vi "SampleRelativeMove.vi"() -> ()   [LabVIEW 2012]
panel:
  in  "Relative Steps":i32=15000
  in  "Motor Number":i32=1
  in  "stop":bool
  out "Position Status":i32
  out "error out":errorcluster
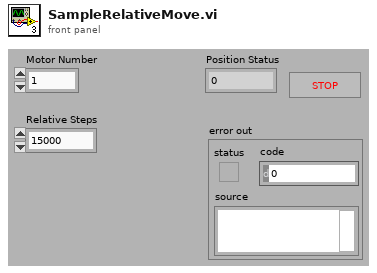
[diagram p1: front panel]
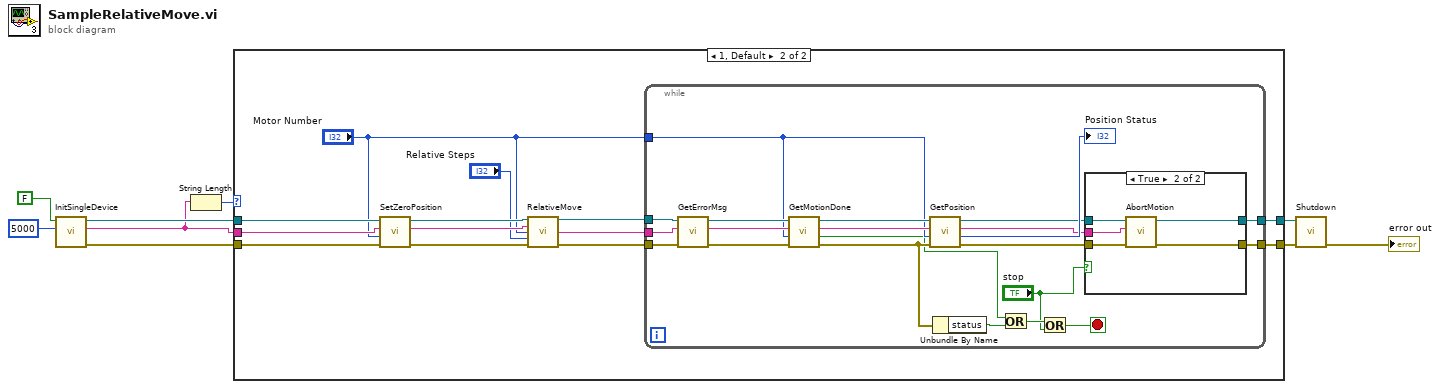
[diagram p0: block diagram]
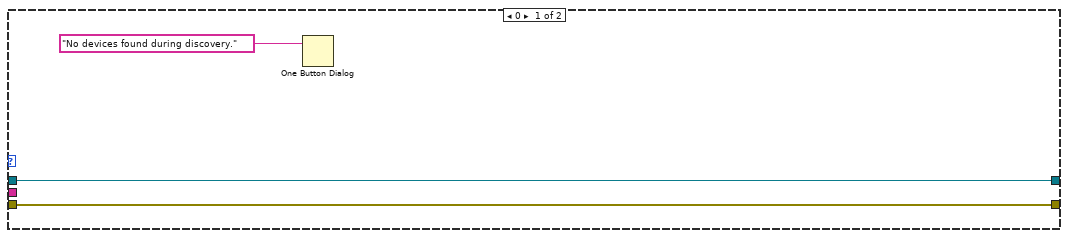
[diagram p2: hidden frame]
diagram:
  n1 = call "InitSingleDevice.vi"("msecDelayForDiscovery"=5000, "logging"=FALSE) -> ("error out"=w1:errorcluster, "DeviceKey Out"=w2:string, "CmdLib Out"=w4:refnum<k24>)  [unwired: 3 in]
  n2 = String Length(string=w2) -> (length=w3:i32)
  n3 = case shown="1, Default" w3 {
    tunnel: [w11 w22] -> w6
    tunnel: [w10 w21] -> w5
    tunnel: w4 -> [w11 w20]
    tunnel: w2 -> [_ w18]
    tunnel: w1 -> [w10 w16]
    frame 0 {
      n4 = One Button Dialog(message="No devices found during discovery.") -> ()  [unwired: 1 in, 1 out]
    }
    frame 1, Default {
      n5 = call "SetZeroPosition.vi"("error in (no error)"=w16, "Motor"="Motor Number", "DeviceKey In"=w18, "CmdLib In"=w20) -> ("error out"=w15:errorcluster, "DeviceKey Out"=w17:string, "CmdLib Out"=w19:refnum<k24>)  [unwired: 1 in]
      n6 = call "RelativeMove.vi"("CmdLib In"=w19, "DeviceKey In"=w17, "Motor"="Motor Number", "Relative Steps"="Relative Steps", "error in (no error)"=w15) -> ("CmdLib Out"=w25:refnum<k24>, "DeviceKey Out"=w24:string, "error out"=w23:errorcluster)  [unwired: 8 in]
      n7 = while {
        tunnel: "Motor Number" -> [w42]
        tunnel: w25 -> [w41]
        tunnel: w24 -> [w40]
        tunnel: w23 -> [w39]
        tunnel: [w27] -> w22
        tunnel: [w29] -> w21
        stop <- w32 stop-if-true
        n8 = call "GetErrorMsg.vi"("error in (no error)"=w39, "DeviceKey In"=w40, "CmdLib In"=w41) -> ("error out"=w38:errorcluster, "DeviceKey Out"=w44:string, "CmdLib Out"=w43:refnum<k24>)  [unwired: 2 in]
        n9 = call "GetMotionDone.vi"("error in (no error)"=w38, "Motor"=w42, "DeviceKey In"=w44, "CmdLib In"=w43) -> ("error out"=w36:errorcluster, "Is Motion Done"=w35:bool, "DeviceKey Out"=w46:string, "CmdLib Out"=w45:refnum<k24>)
        n10 = call "GetPosition.vi"("error in (no error)"=w36, "Motor"=w42, "DeviceKey In"=w46, "CmdLib In"=w45) -> ("error out"=w30:errorcluster, "Position"=→"Position Status":i32, "DeviceKey Out"=w26:string, "CmdLib Out"=w28:refnum<k24>)
        n11 = Unbundle By Name(w36) -> ("status"=w37:bool)
        n12 = Or(x=w35, y=w37) -> (x .or. y?=w33:bool)
        n13 = Or(x=w33, y="stop") -> (x .or. y?=w32:bool)
        n14 = case shown="True" "stop" {
          tunnel: w30 -> [w47 w53]
          tunnel: [w47 w52] -> w29
          tunnel: w28 -> [w48 w51]
          tunnel: [w48 w50] -> w27
          tunnel: w26 -> [_ w49]
          frame False {
          }
          frame True {
            n15 = call "AbortMotion.vi"("error in (no error)"=w53, "DeviceKey In"=w49, "CmdLib In"=w51) -> ("error out"=w52:errorcluster, "CmdLib Out"=w50:refnum<k24>)  [unwired: 2 in, 1 out]
          }
        }
      }
    }
  }
  n16 = call "Shutdown.vi"("error in (no error)"=w5, "CmdLib In"=w6) -> ("error out"=→"error out":errorcluster)  [unwired: 4 in, 1 out]
